vi "HTTP Get Helper.vi"(7 "Arguments":string[](array[string]), 8 "Error In":errorcluster, 10 "JSON Request":string, 11 "XBMC Ref":T1) -> (0 "Error Out":errorcluster, 1 "Response":string, 3 "XBMC Ref":T1)   [LabVIEW 2013, in "LMH-Kodi.lvlib"]
uses:
  LMH-Kodi.lvlib
  Type Defs/XBMC Ref.ctl
  <vilib>/httpClient/ClientHandle.ctl
  <vilib>/httpClient/LabVIEWHTTPClient.lvlib
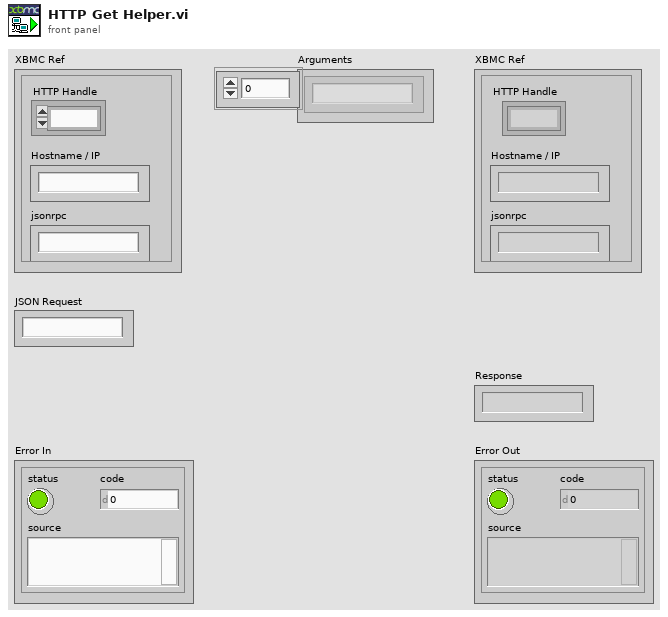
[diagram p1: front panel]
types:
  T1 = typedef "LMH-Kodi.lvlib/XBMC Ref.ctl" = cluster{"HTTP Handle":T2, "Hostname / IP":string, "jsonrpc":string}
  T2 = typedef "LabVIEWHTTPClient.lvlib/ClientHandle.ctl" = refnum<k1>
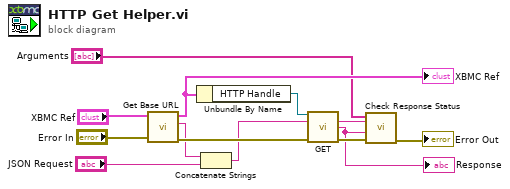
[diagram p0: block diagram]
diagram:
  n1 = call "Get Base URL.vi"("Error In"="Error In", "XBMC Ref"="XBMC Ref") -> ("Error Out"=w11:errorcluster, "XBMC JSON Base URL"=w7:string, "XBMC Ref"=w10:T1)  [unwired: 7 in]
  "XBMC Ref" <- w10
  n2 = Unbundle By Name(w10) -> ("HTTP Handle"=w9:T2)
  n3 = Concatenate Strings(w7, "JSON Request") -> (w8:string)
  n4 = call <vilib>:"GET.vi"("client handle"=w9, "url"=w8, "error in (no error)"=w11) -> ("headers"=w5:string, "body"=w1:string, "error out"=w6:errorcluster)  [unwired: 9 in, 1 out]
  "Response" <- w1
  n5 = call "Check Response Status.vi"("Error In"=w6, "Body"=w1, "Headers"=w5, "Arguments"="Arguments") -> ("Error Out"=→"Error Out":errorcluster)  [unwired: 7 in]
